vi "SimAdc Initialize Virtual Channels.vi"(8 "error in":errorcluster, 11 "simadc in":T1) -> (0 "error out":errorcluster, 2 "channel identifiers":string[](array[string]), 3 "simadc out":T1)   [LabVIEW 2013]
doc: "Initiates simulated ADC, returns simulated channels descriptors."
uses:
  SimAdc Config.ctl
  SimAdc Channel Cfg.ctl
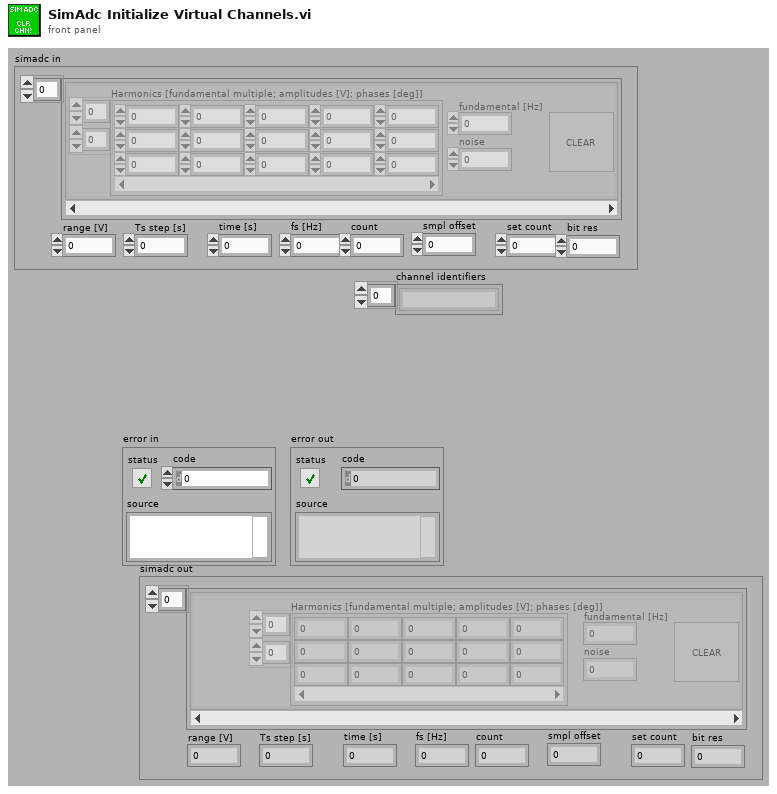
[diagram p1: front panel]
types:
  T1 = typedef "SimAdc Config.ctl" = cluster{"channels":T2[], "range [V]":dbl, "Ts step [s]":dbl, "time [s]":dbl, "fs [Hz]":dbl, "count":i64, "smpl offset":i64, "set count":i64, "bit res":i32}
  T2 = typedef "SimAdc Channel Cfg.ctl" = cluster{"harmonics":dbl[][], "btn clear":bool, "noise":dbl, "fundamental [Hz]":dbl}
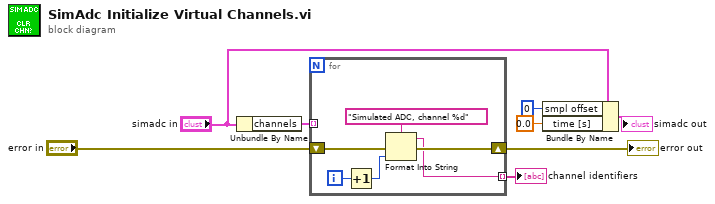
[diagram p0: block diagram]
diagram:
  n1 = Unbundle By Name("simadc in") -> ("channels"=w8:T2[])
  n2 = for {
    shift-right: [w13] -> w6
    shift-left: "error in" -> [w14]
    tunnel: w8 -> [_] mode=indexing
    tunnel: [w9] -> w2 mode=indexing
    i -> [w12]
    n3 = Increment(x=w12) -> (x+1=w11:i32)
    n4 = Format Into String(format string="Simulated ADC, channel %d", error in=w14, w11) -> (resulting string=w9:string, error out=w13:errorcluster)  [unwired: 1 in]
  }
  "error out" <- w6
  "channel identifiers" <- w2
  n5 = Bundle By Name(cluster="simadc in", "smpl offset"=i64 0, "time [s]"=0.0) -> (→"simadc out":T1)
